vi "Verify Git.vi"(8 "error in (no error)":errorcluster, 11 "Git in":refnum<class "Git.lvclass">) -> (0 "error out":errorcluster, 3 "Git out":refnum<class "Git.lvclass">)   [LabVIEW 2019, in "Git.lvclass"]
uses:
  Git.lvclass
  <vilib>/Platform/browser.llb/Open URL in Default Browser (string).vi
panel:
  out "standard error":string
  out "standard output":string
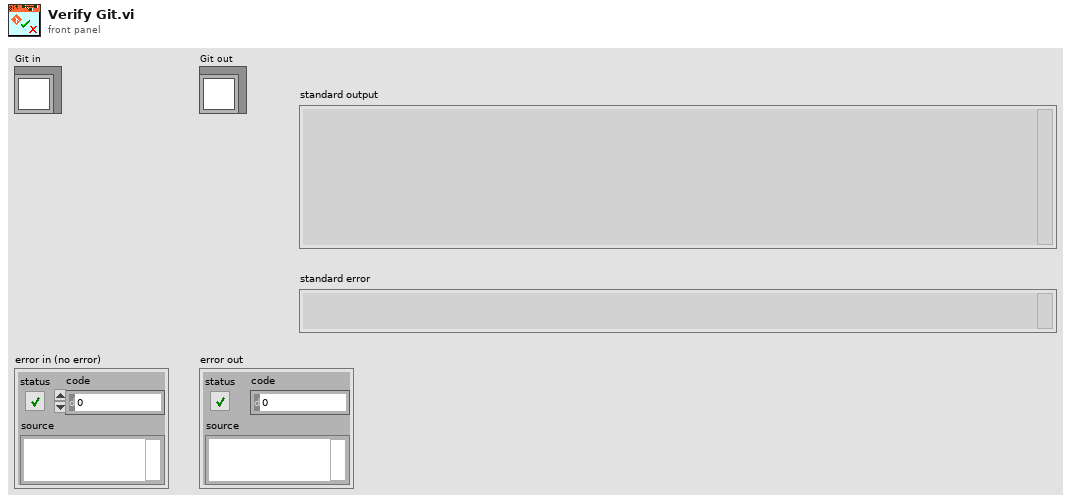
[diagram p1: front panel]
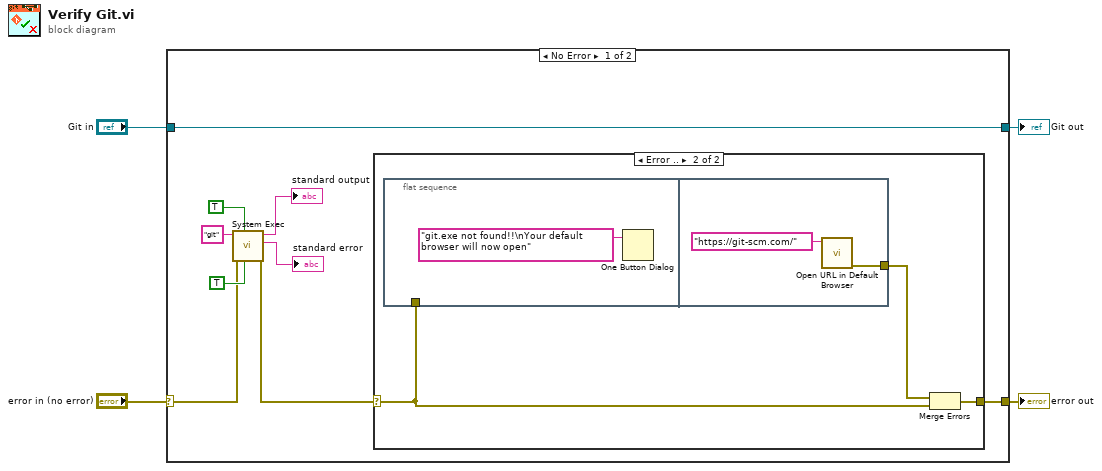
[diagram p0: block diagram]
diagram:
  n1 = case shown="No Error" "error in (no error)" {
    selector: "error in (no error)" -> [w9 w22]
    tunnel: "Git in" -> [w13 w21]
    tunnel: [w5 w22] -> w3
    tunnel: [w13 w21] -> w2
    frame No Error {
      n2 = call <vilib>:"System Exec.vi"("run minimized? (F)"=TRUE, "wait until completion? (T)"=TRUE, "error in (no error)"=w9, "command line"="git") -> ("error out"=w6:errorcluster, "standard error"=→"standard error":string, "standard output"=→"standard output":string)  [unwired: 4 in, 1 out]
      n3 = case shown="Error .." w6 {
        selector: w6 -> [w14 w16]
        tunnel: [w14 w15] -> w5
        frame No Error {
        }
        frame Error {
          n4 = flat-sequence {
            tunnel: w16 -> [_]
            tunnel: [w19] -> w17
            frame #0 {
              n5 = One Button Dialog(message="git.exe not found!!\nYour default browser will now open") -> ()  [unwired: 1 in, 1 out]
            }
            frame #1 {
              n6 = call-poly <vilib>:"Open URL in Default Browser.vi"("URL"="https://git-scm.com/") -> ("error out"=w19:errorcluster)  [unwired: 5 in, 1 out]
            }
          }
          n7 = Merge Errors(w17, w16) -> (w15:errorcluster)
        }
      }
    }
    frame Error {
    }
  }
  "Git out" <- w2
  "error out" <- w3
